vi "getValueFromXMLNative.vi"(8 "error in (no error)":errorcluster, 10 "eventXML":refnum<k20>, 11 "SingleToneRamp in":refnum<class "SingleToneRamp.lvclass">) -> (0 "error out":errorcluster, 2 "eventXML out":refnum<k20>, 3 "SingleToneRamp out":refnum<class "SingleToneRamp.lvclass">)   [LabVIEW 2011, in "Tools.lvlib" / "Scripting.lvlib" / "SingleToneRamp.lvclass"]
uses:
  SingleToneRamp.lvclass
  <vilib>/xml/Close Reference(Node).vi
  <vilib>/xml/NI_XML.lvlib
  ScriptEvent.lvclass
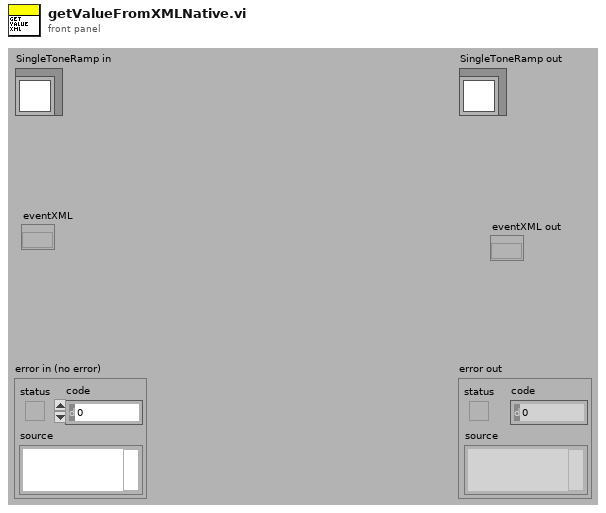
[diagram p1: front panel]
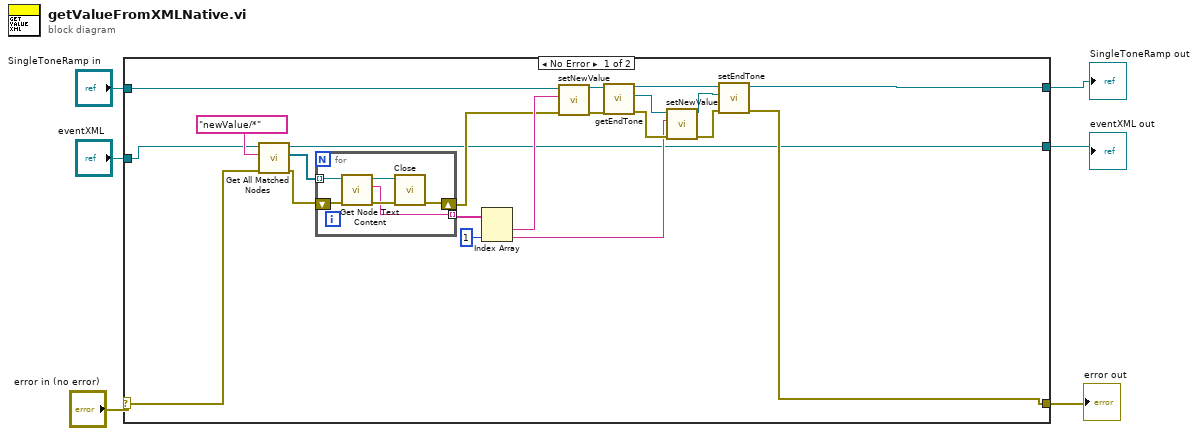
[diagram p0: block diagram]
diagram:
  n1 = case shown="No Error" "error in (no error)" {
    selector: "error in (no error)" -> [w21 w34]
    tunnel: [w9 w34] -> w5
    tunnel: [w18 w35] -> w4
    tunnel: "SingleToneRamp in" -> [w19 w35]
    tunnel: "eventXML" -> [w22 _]
    tunnel: [w8 _] -> w1
    frame No Error {
      n2 = call <vilib>:"Get All Matched Nodes.vi"("error in (no error)"=w21, "XPath expression"="newValue/*", "node in"=w22) -> ("error out"=w27:errorcluster, "node result array"=w25:refnum<k20>[], "node out"=w8:refnum<k20>)  [unwired: 6 in]
      n3 = for {
        tunnel: w25 -> [w30] mode=indexing
        tunnel: [w29] -> w24 mode=indexing
        shift-right: [w28] -> w10
        shift-left: w27 -> [w31]
        n4 = call <vilib>:"Get Node Text Content.vi"("error in (no error)"=w31, "node in"=w30) -> ("error out"=w32:errorcluster, "node text"=w29:string, "node out"=w33:refnum<k20>)  [unwired: 7 in]
        n5 = call-poly <vilib>:"Close.vi"("error in (no error)"=w32, "node"=w33) -> ("error out"=w28:errorcluster)  [unwired: 7 in]
      }
      n6 = Index Array(array=w24, index #2=1 ("index")) -> (element #1=w11:string, element #2=w12:string)  [unwired: 1 in]
      n7 = call "setNewValue.vi"("error in (no error)"=w10, "newValue"=w11, "ScriptEvent.lvclass in"=w19) -> ("error out"=w20:errorcluster, "ScriptEvent.lvclass out"=w14:refnum<class "SingleToneRamp.lvclass">)  [unwired: 7 in]
      n8 = call "getEndTone.vi"("error in (no error)"=w20, "SingleToneRamp.lvclass in"=w14) -> ("error out"=w13:errorcluster, "endTone"=w7:refnum<class "SingleTone.lvclass">, "SingleToneRamp.lvclass out"=w15:refnum<class "SingleToneRamp.lvclass">)  [unwired: 7 in]
      n9 = call "setNewValue.vi"("error in (no error)"=w13, "newValue"=w12, "ScriptEvent.lvclass in"=w7) -> ("error out"=w17:errorcluster, "ScriptEvent.lvclass out"=w16:refnum<class "SingleTone.lvclass">)  [unwired: 7 in]
      n10 = call "setEndTone.vi"("error in (no error)"=w17, "EndTone"=w16, "SingleToneRamp.lvclass in"=w15) -> ("error out"=w9:errorcluster, "SingleToneRamp.lvclass out"=w18:refnum<class "SingleToneRamp.lvclass">)  [unwired: 7 in]
    }
    frame Error {
    }
  }
  "error out" <- w5
  "SingleToneRamp out" <- w4
  "eventXML out" <- w1
